vi "Unflatten.vi"(8 "error in (no error)":errorcluster, 11 "Wavelength PEM and Digikröm in":refnum<class "Wavelength PEM and Digikröm.lvclass">) -> (0 "error out":errorcluster, 3 "Wavelength PEM and Digikröm out":refnum<class "Wavelength PEM and Digikröm.lvclass">)   [LabVIEW 2017, in "Wavelength PEM and Digikröm.lvclass"]
uses:
  Global/File Locations.vi
  Scanner/Scanner.lvclass
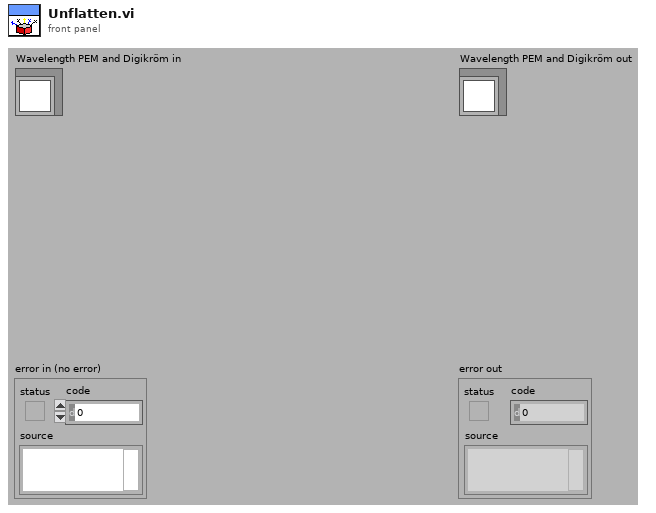
[diagram p1: front panel]
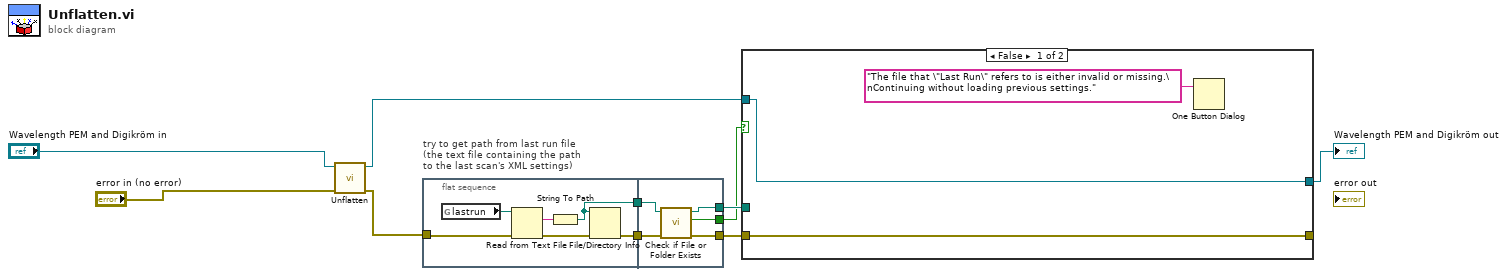
[diagram p0: block diagram]
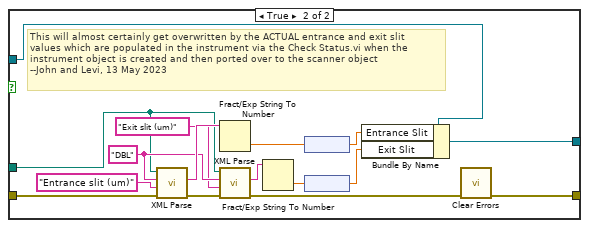
[diagram p2: hidden frame]
diagram:
  n1 = call-parent "Unflatten.vi"("error in (no error)"="error in (no error)", "Scanner in"="Wavelength PEM and Digikröm in") -> ("error out"=w1:errorcluster, "Scanner out"=w3:refnum<class "Wavelength PEM and Digikröm.lvclass">)  [unwired: 8 in]
  n2 = flat-sequence "try to get path from last run file\n(the text file containing the path\nto the last scan's XML settings)" {
    tunnel: [w16] -> w8
    tunnel: [w12] -> w7
    tunnel: w1 -> [w11]
    tunnel: [w20] -> w6
    tunnel: [w21] -> w5
    tunnel: w8 -> [w18]
    tunnel: w7 -> [w19]
    tunnel: [w17] -> w4
    frame #0 {
      n3 = global read "File Locations.vi" "lastrun"() -> (w14:path)
      n4 = Read from Text File(file (use dialog)=w14, error in=w11) -> (text=w15:string, error out=w13:errorcluster)  [unwired: 4 out]
      n5 = String To Path(string=w15) -> (path=w16:path)
      n6 = File/Directory Info(path=w16, error in=w13) -> (error out=w12:errorcluster)  [unwired: 6 out]
    }
    frame #1 {
      n7 = call <vilib>:"Check if File or Folder Exists.vi"("error in (no error)"=w19, "path"=w18) -> ("error out"=w20:errorcluster, "file or folder exists?"=w17:bool, "dup path"=w21:path)  [unwired: 7 in]
    }
  }
  n8 = case shown="False" w4 {
    tunnel: [w22 w40] -> w2
    tunnel: w6 -> [w23 w39]
    tunnel: w5 -> [_ w32]
    tunnel: [w23 w37] -> _
    tunnel: w3 -> [w22 w25]
    frame False {
      n9 = One Button Dialog(message="The file that \"Last Run\" refers to is either invalid or missing.\nContinuing without loading previous settings.") -> ()  [unwired: 1 in, 1 out]
    }
    frame True {
      w33 = "DBL"
      # "This will almost certainly get overwritten by the ACTUAL entrance and exit slit \nvalues which are populated in the instrument via the Check Status.vi when the \ninstrument object is created and then ported over to the scanner object\n--John and Levi, 13 May 2023"
      n10 = call "XML Parse.vi"("error in (no error)"=w39, "Name String"="Entrance slit (um)", "Type String"=w33, "Path"=w32) -> ("error out"=w30:errorcluster, "String Out"=w36:string)  [unwired: 6 in]
      n11 = Fract/Exp String To Number(string=w36) -> (number=w34:dbl)  [unwired: 3 in, 1 out]
      n12 = call "XML Parse.vi"("error in (no error)"=w30, "Name String"="Exit slit (um)", "Type String"=w33, "Path"=w32) -> ("error out"=w26:errorcluster, "String Out"=w29:string)  [unwired: 6 in]
      n13 = Fract/Exp String To Number(string=w29) -> (number=w28:dbl)  [unwired: 3 in, 1 out]
      n14 = node(w34) -> (w35:dbl[unit])
      n15 = node(w28) -> (w27:dbl[unit])
      n16 = Bundle By Name(cluster=w25, "Entrance Slit"=w35, "Exit Slit"=w27) -> (w40:refnum<class "Wavelength PEM and Digikröm.lvclass">)
      n17 = call <vilib>:"Clear Errors.vi"("error in (no error)"=w26) -> ("error out"=w37:errorcluster)  [unwired: 5 in, 1 out]
    }
  }
  "Wavelength PEM and Digikröm out" <- w2
